vi "Test Unnamed Clusters to JSON Arrays.vi"() -> ()   [LabVIEW 2017]
uses:
  JSONtext.lvlib
panel:
  out "<JSON>":string
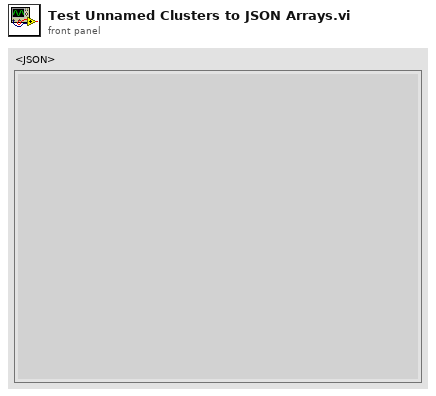
[diagram p1: front panel]
types:
  T1 = cluster{cluster{"Name":string, "<JSON>Config":string}, "<JSON>":string}
  T2 = cluster{cluster{string, "<JSON>":string, i32}, cluster{cluster{"Name":string, "<JSON>Config":string}, "<JSON>":string}}
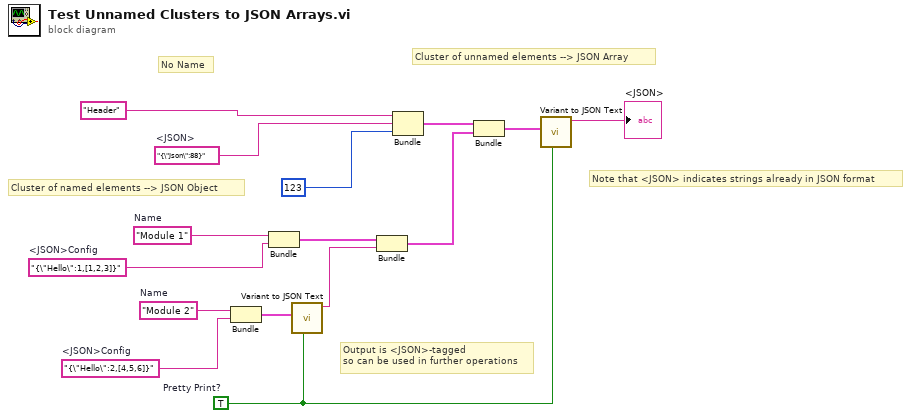
[diagram p0: block diagram]
diagram:
  w6 = "{\"Hello\":1,[1,2,3]}"  # <JSON>Config
  w7 = "{\"Hello\":2,[4,5,6]}"  # <JSON>Config
  w8 = "Module 2"  # Name
  w9 = "Module 1"  # Name
  w1 = TRUE  # Pretty Print?
  w11 = "{\"Json\":88}"  # <JSON>
  # "Output is <JSON>-tagged\nso can be used in further operations"
  # "Cluster of named elements --> JSON Object"
  # "Cluster of unnamed elements --> JSON Array"
  # "No Name"
  # "Note that <JSON> indicates strings already in JSON format"
  n1 = Bundle("Name"=w8, "<JSON>Config"=w7) -> (w3:cluster{"Name":string, "<JSON>Config":string})  [unwired: 1 in]
  n2 = Bundle("Name"=w9, "<JSON>Config"=w6) -> (w10:cluster{"Name":string, "<JSON>Config":string})  [unwired: 1 in]
  n3 = call "Variant to JSON Text.vi"("Pretty Print?"=w1, "Variant"=w3) -> ("<JSON>"=w2:string)  [unwired: 7 in, 2 out]
  n4 = Bundle(w10, "<JSON>"=w2) -> (w5:T1)  [unwired: 1 in]
  n5 = Bundle("Header", "<JSON>"=w11, 123) -> (w15:cluster{string, "<JSON>":string, i32})  [unwired: 1 in]
  n6 = Bundle(w15, w5) -> (w14:T2)  [unwired: 1 in]
  n7 = call "Variant to JSON Text.vi"("Pretty Print?"=w1, "Variant"=w14) -> ("<JSON>"=→"<JSON>":string)  [unwired: 7 in, 2 out]
